vi "RSNRPZ Fetch Measurement.vi"(8 "error in (no error)":errorcluster, 10 "Channel (1)":i32=1, 11 "VISA session":refnum<visa-resource-name> caption="VISA resource name") -> (0 "error out":errorcluster, 2 "Measurement":dbl format="%.3p", 3 "dup VISA session":refnum<visa-resource-name> caption="VISA resource name")   [LabVIEW 2019]
doc: "This VI returns the measurement the sensor acquires for the channel you specify. The measurement is from an acquisition that you previously initiated. \n\nYou use the RSNRPZ Initiate.vi to start an acquisition on the channels that you specify. You use the RSNRPZ Get Measurement Complete State.vi to determine when the acquisition is complete.\n\nYou can call the RSNRPZ Read Measurement.vi instead of the RSNRPZ Initiate.vi. The RSNRPZ Read Measurement.vi starts an acquisition, waits for the acquisition to complete, and returns the measurement for the channel you specify.\n\nNote:\n\n1) If the measurement is not available, acquistion has not been initialized or it's still in progress function retrune an error (0xBFFC0100 Measurement is not available)"
uses:
  rsnrpz_32.dll
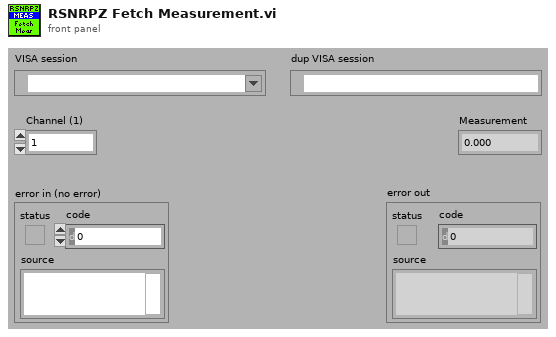
[diagram p1: front panel]
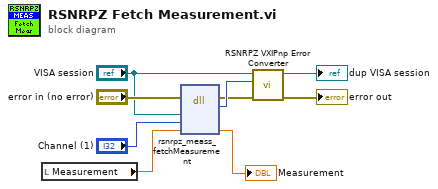
[diagram p0: block diagram]
diagram:
  n1 = local read "Measurement"() -> (w7:dbl)
  n2 = dll-call lib="C:/Users/LABadmin/Documents/Jarvis/user_lib/rsnrpz/rsnrpz_32.dll" fn="rsnrpz_meass_fetchMeasurement"(error in="error in (no error)", "Instrument Handle"="VISA session", "Channel"="Channel (1)", "Measurement"=w7) -> (error out=w5:errorcluster, "Status"=w9:i32, "Measurement"=→"Measurement":dbl)  [unwired: 4 in, 1 out]
  n3 = call <instrlib>:"RSNRPZ VXIPnp Error Converter.vi"("error in"=w5, "VXIPnp error code"=w9, "VISA session"="VISA session") -> ("error out"=→"error out":errorcluster, "dup VISA session"=→"dup VISA session":refnum<visa-resource-name>)  [unwired: 7 in]
